vi "TimeSyncServer_Execute.vi"(8 "error in (no error)":errorcluster) -> ()   [LabVIEW 2019, in "PhotonVisionLib.lvlib"]
doc: "Create a new TargetCorner data cluster\n\nInputs:\n - X -- \n - Y -- \n\nOutputs:\n - TargetCorner -- Created TargetCorner cluster."
uses:
  PhotonVisionLib.lvlib
  <vilib>/Rock Robotics/WPI/ThirdParty/JAS_Junk/TrajLib/Trajectory_Library.lvlib
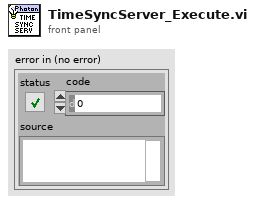
[diagram p1: front panel]
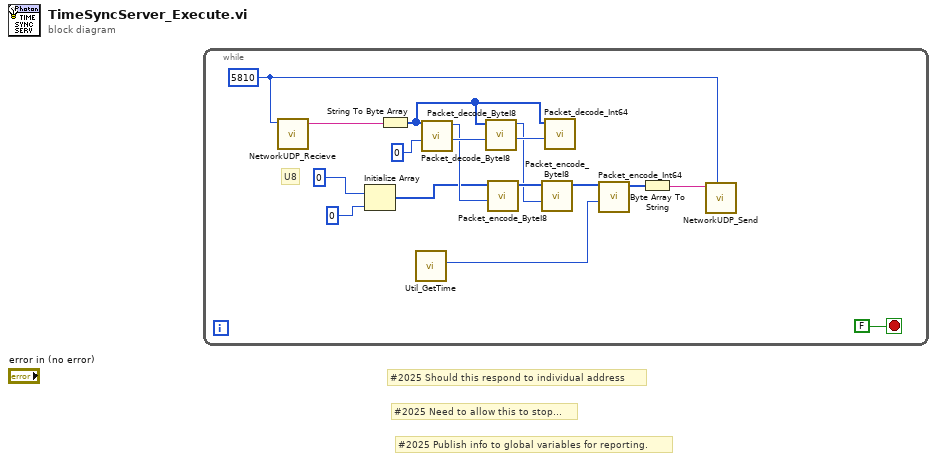
[diagram p0: block diagram]
diagram:
  # "#2025 Publish info to global variables for reporting."
  # "#2025 Need to allow this to stop..."
  # "#2025 Should this respond to individual address"
  n1 = while {
    stop <- FALSE stop-if-true
    w6 = u16 5810 ("receiver port")
    # "U8"
    n2 = call <vilib>:"NetworkUDP_Recieve.vi"("receiver port"=w6) -> ("data out"=w16:string)  [unwired: 7 in, 3 out]
    n3 = Initialize Array(u8 0 ("element"), 0 ("dimension size")) -> (w1:u8[])
    n4 = String To Byte Array(string=w16) -> (unsigned byte array=w14:u8[])
    n5 = call <vilib>:"Util_GetTime.vi"() -> ("FPGA_Time_MicroSeconds"=w7:u64)  [unwired: 9 in, 2 out]
    n6 = call "Packet_decode_ByteI8.vi"("StartByte"=0, "RawData"=w14) -> ("NextByte"=w13:i32, "Int8_Value"=w9:i8)  [unwired: 8 in]
    n7 = call "Packet_decode_ByteI8.vi"("StartByte"=w13, "RawData"=w14) -> ("NextByte"=w12:i32, "Int8_Value"=w8:i8)  [unwired: 8 in]
    n8 = call "Packet_encode_ByteI8.vi"("Int8_Value"=w9, "RawData In"=w1) -> ("RawData Out"=w11:u8[])  [unwired: 9 in]
    n9 = call "Packet_encode_ByteI8.vi"("Int8_Value"=w8, "RawData In"=w11) -> ("RawData Out"=w10:u8[])  [unwired: 9 in]
    n10 = call "Packet_decode_Int64.vi"("StartByte"=w12, "RawData"=w14) -> ()  [unwired: 8 in, 2 out]
    n11 = call "Packet_encode_Int64.vi"("Int64_Value"=w7, "RawData In"=w10) -> ("RawData Out"=w5:u8[])  [unwired: 9 in]
    n12 = Byte Array To String(unsigned byte array=w5) -> (string=w4:string)
    n13 = call <vilib>:"NetworkUDP_Send.vi"("remote port"=w6, "data string"=w4) -> ()  [unwired: 7 in, 3 out]
  }
